vi "APS set point table2.vi"(7 "Point":T1, 8 "error in (no error)":errorcluster caption="错误输入（无错误）", 9 "Index":i32, 10 "Axis_ID_Array":i32, 11 "Dimension":i32) -> (0 "error out":errorcluster caption="错误输出", 2 "Axis_ID_Array out":i32, 3 "function return":i32, 5 "Point out":T1)   [LabVIEW 2011, in "APS168.lvlib"]
doc: "I32 FNTYPE APS_set_point_table2( I32 Dimension, I32 *Axis_ID_Array, I32 Index, POINT_DATA2 *Point );"
uses:
  APS168.lvlib
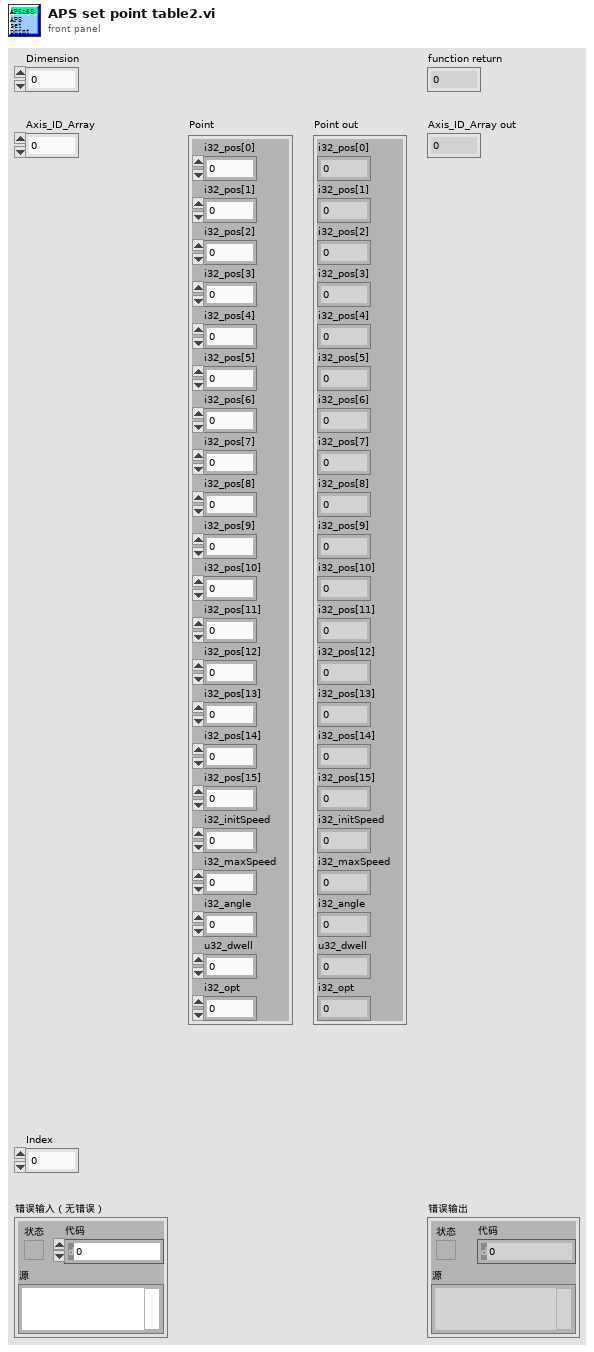
[diagram p1: front panel]
types:
  T1 = cluster{"i32_pos[0]":i32, "i32_pos[1]":i32, "i32_pos[2]":i32, "i32_pos[3]":i32, "i32_pos[4]":i32, "i32_pos[5]":i32, "i32_pos[6]":i32, "i32_pos[7]":i32, "i32_pos[8]":i32, "i32_pos[9]":i32, "i32_pos[10]":i32, "i32_pos[11]":i32, "i32_pos[12]":i32, "i32_pos[13]":i32, "i32_pos[14]":i32, "i32_pos[15]":i32, "i32_initSpeed":i32, "i32_maxSpeed":i32, "i32_angle":i32, "u32_dwell":u32, "i32_opt":i32}
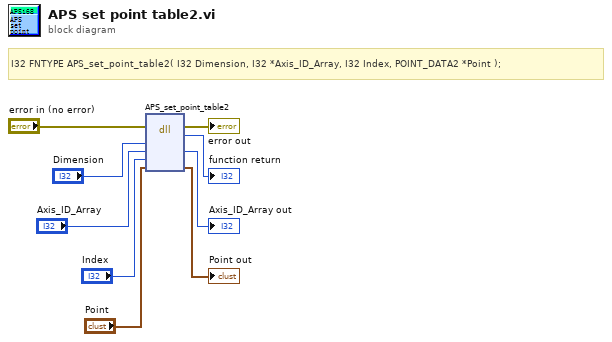
[diagram p0: block diagram]
diagram:
  # "I32 FNTYPE APS_set_point_table2( I32 Dimension, I32 *Axis_ID_Array, I32 Index, POINT_DATA2 *Point );"
  n1 = dll-call lib="PTH1Labs E软件ADLINK 204CAPS_1_7_1_LIB line 连续运动204APS168.*" fn="APS_set_point_table2"(error in="error in (no error)", "Dimension"="Dimension", "Axis_ID_Array"="Axis_ID_Array", "Index"="Index", "Point"="Point") -> (error out=→"error out":errorcluster, →"function return":i32, "Axis_ID_Array"=→"Axis_ID_Array out":i32, "Point"=→"Point out":T1)  [unwired: 4 in, 1 out]
